vi "MB Slave Read All Discrete Inputs (poly).vi"(5 "error in":errorcluster) -> (15 "Discrete Inputs":bool[](array[boolean]), 19 "error out":errorcluster)   [LabVIEW 2020]
doc: "Reads all discrete inputs from the slave's memory table."
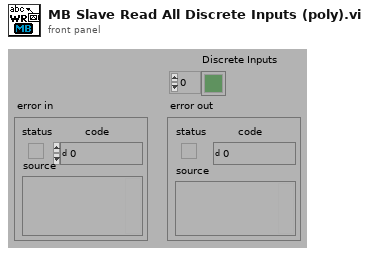
[diagram p1: front panel]
types:
  T1 = enum16{"Discrete Inputs", "Coils", "Input Registers", "Holding Registers"}
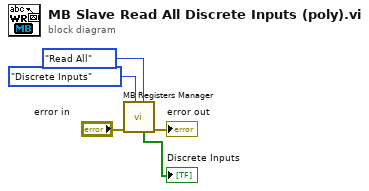
[diagram p0: block diagram]
diagram:
  n1 = call "MB Registers Manager.vi"("Function"=enum16{"Init", "Read", "Write", "Read All"}."Read All", "Table"=T1."Discrete Inputs", "error in (no error)"="error in") -> ("error out"=→"error out":errorcluster, "Bits out"=→"Discrete Inputs":bool[])  [unwired: 4 in, 3 out]
